vi "Arm_Pos_Begin.vi"   [LabVIEW 2020]
uses:
  Robot Global Data.vi
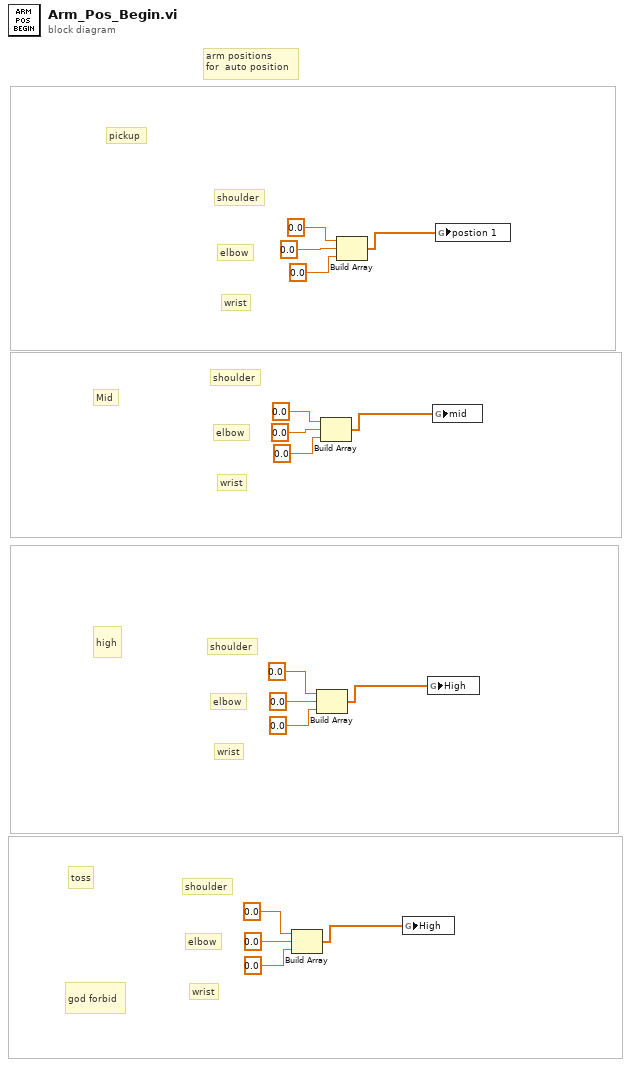
[diagram p0: block diagram]
diagram:
  # "arm positions\nfor  auto position"
  # "god forbid"
  # "wrist"
  # "elbow"
  # "shoulder"
  # "toss"
  # "wrist"
  # "elbow"
  # "shoulder"
  # "wrist"
  # "elbow"
  # "shoulder"
  # "wrist"
  # "elbow"
  # "shoulder"
  # "high"
  # "Mid"
  # "pickup"
  n1 = Build Array(0.0 ("element"), 0.0 ("element"), 0.0 ("element")) -> (w16:dbl[])
  n2 = Build Array(0.0 ("element"), 0.0 ("element"), 0.0 ("element")) -> (w9:dbl[])
  n3 = Build Array(0.0 ("element"), 0.0 ("element"), 0.0 ("element")) -> (w8:dbl[])
  n4 = Build Array(0.0 ("element"), 0.0 ("element"), 0.0 ("element")) -> (w1:dbl[])
  n5 = global write "Robot Global Data.vi" "High"(w16) -> ()
  n6 = global write "Robot Global Data.vi" "High"(w9) -> ()
  n7 = global write "Robot Global Data.vi" "mid"(w8) -> ()
  n8 = global write "Robot Global Data.vi" "postion 1"(w1) -> ()
